vi "arduinoSendCommand.vi"(4 "Wait For Completion":bool=TRUE, 6 "Input Command":string, 7 "error in (no error)":errorcluster, 9 "Input Recieve Log":string, 10 "VISA resource name":refnum<visa-resource-name>) -> (0 "error out":errorcluster, 1 "Command Accepted":bool, 2 "Output Recieve Log":string, 3 "VISA resource name out":refnum<visa-resource-name>)   [LabVIEW 2019]
panel:
  out "Command Rejected":bool
  in  "Wait For Acceptance":bool=TRUE
  out "Command Root":string
  in  "millisecond timer value":u32=200
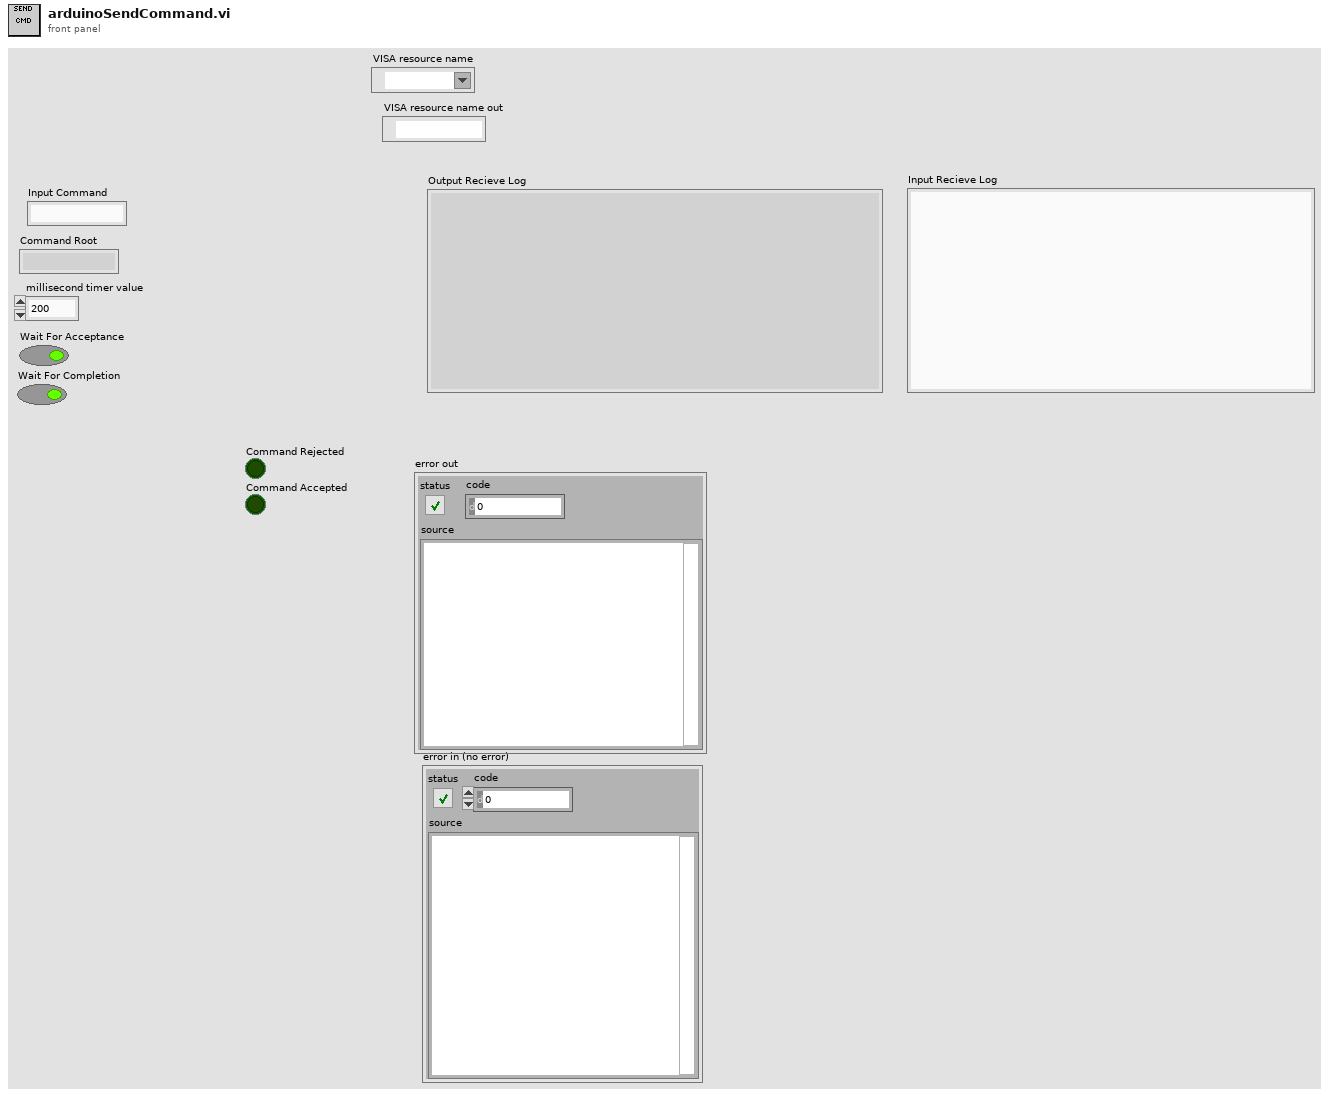
[diagram p1: front panel]
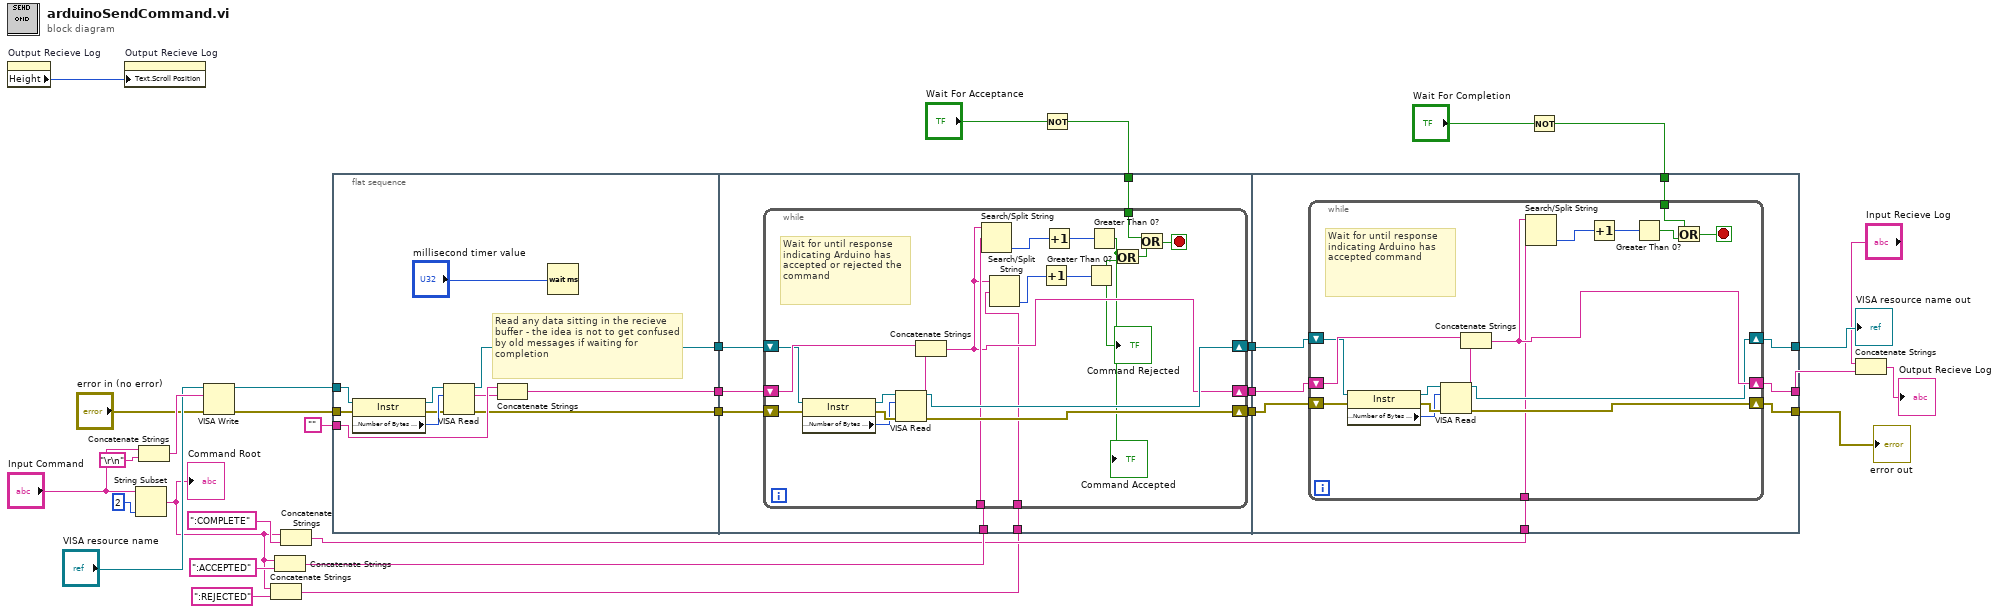
[diagram p0: block diagram]
diagram:
  n1 = property on="Output Recieve Log" class="Str"() -> ("Height"=w30:u32)  [unwired: 2 in, 2 out]
  n2 = property on="Output Recieve Log" class="Str"("Text.Scroll Position"=w30) -> ()  [unwired: 2 in, 2 out]
  n3 = String Subset(string="Input Command", length (rest)=2 ("length (rest)")) -> (substring=w3:string)  [unwired: 1 in]
  "Command Root" <- w3
  n4 = Concatenate Strings("Input Command", "\r\n") -> (w29:string)
  n5 = VISA Write(VISA resource name="VISA resource name", write buffer=w29, error in (no error)="error in (no error)") -> (VISA resource name out=w32:refnum<visa-resource-name>, error out=w31:errorcluster)  [unwired: 1 out]
  n6 = Concatenate Strings(w3, ":REJECTED" ("string")) -> (w1:string)
  n7 = Concatenate Strings(w3, ":ACCEPTED" ("string")) -> (w5:string)
  n8 = Concatenate Strings(w3, ":COMPLETE" ("string")) -> (w4:string)
  n9 = flat-sequence {
    tunnel: w31 -> [w41]
    tunnel: w32 -> [w42]
    tunnel: "" -> [w40]
    tunnel: [w35] -> w27
    tunnel: [w33] -> w13
    tunnel: [w37] -> w12
    tunnel: w27 -> [w50]
    tunnel: w5 -> [w48]
    tunnel: [w52] -> w21
    tunnel: [w51] -> w20
    tunnel: [w49] -> w19
    tunnel: w13 -> [w46]
    tunnel: w12 -> [w47]
    tunnel: w7 -> [w45]
    tunnel: w1 -> [w44]
    tunnel: [w74] -> w10
    tunnel: [w77] -> w23
    tunnel: [w80] -> w24
    tunnel: w21 -> [w81]
    tunnel: w20 -> [w78]
    tunnel: w19 -> [w79]
    tunnel: w6 -> [w76]
    tunnel: w4 -> [w75]
    frame #0 {
      # "Read any data sitting in the recieve buffer - the idea is not to get confused by old messages if waiting for completion"
      n10 = property class="Instr"(reference=w42, error in=w41) -> (reference out=w38:refnum<visa-resource-name>, error out=w34:errorcluster, "Serial Settings:Number of Bytes at Serial Port"=w36:u32)
      n11 = VISA Read(VISA resource name=w38, byte count=w36, error in (no error)=w34) -> (VISA resource name out=w37:refnum<visa-resource-name>, read buffer=w39:string, error out=w33:errorcluster)  [unwired: 1 out]
      n12 = Concatenate Strings(w40, w39) -> (w35:string)
      n13 = Wait (ms)(milliseconds to wait="millisecond timer value") -> ()  [unwired: 1 out]
    }
    frame #1 {
      n14 = while {
        shift-right: [w64] -> w51
        shift-left: w47 -> [w69]
        shift-right: [w65] -> w52
        shift-left: w46 -> [w67]
        shift-right: [w61] -> w49
        shift-left: w50 -> [w72]
        tunnel: w48 -> [w62]
        tunnel: w45 -> [w56]
        tunnel: w44 -> [w60]
        stop <- w53 stop-if-true
        # "Wait for until response indicating Arduino has accepted or rejected the command"
        n15 = property class="Instr"(reference=w69, error in=w67) -> (reference out=w68:refnum<visa-resource-name>, error out=w66:errorcluster, "Serial Settings:Number of Bytes at Serial Port"=w63:u32)
        n16 = VISA Read(VISA resource name=w68, byte count=w63, error in (no error)=w66) -> (VISA resource name out=w64:refnum<visa-resource-name>, read buffer=w73:string, error out=w65:errorcluster)  [unwired: 1 out]
        n17 = Concatenate Strings(w72, w73) -> (w61:string)
        n18 = Search/Split String(string=w61, search string/char (-)=w62) -> (offset of match=w71:i32)  [unwired: 1 in, 2 out]
        n19 = Search/Split String(string=w61, search string/char (-)=w60) -> (offset of match=w59:i32)  [unwired: 1 in, 2 out]
        n20 = Increment(x=w59) -> (x+1=w58:i32)
        n21 = Increment(x=w71) -> (x+1=w70:i32)
        n22 = Greater Than 0?(x=w58) -> (x > 0?=w54:bool)
        "Command Rejected" <- w54
        n23 = Greater Than 0?(x=w70) -> (x > 0?=w57:bool)
        "Command Accepted" <- w57
        n24 = Or(x=w57, y=w54) -> (x .or. y?=w55:bool)
        n25 = Or(x=w56, y=w55) -> (x .or. y?=w53:bool)
      }
    }
    frame #2 {
      n26 = while {
        shift-right: [w86] -> w77
        shift-left: w78 -> [w91]
        shift-right: [w87] -> w80
        shift-left: w81 -> [w89]
        shift-right: [w93] -> w74
        shift-left: w79 -> [w96]
        tunnel: w76 -> [w83]
        tunnel: w75 -> [w82]
        stop <- w92 stop-if-true
        # "Wait for until response indicating Arduino has accepted command"
        n27 = property class="Instr"(reference=w91, error in=w89) -> (reference out=w90:refnum<visa-resource-name>, error out=w88:errorcluster, "Serial Settings:Number of Bytes at Serial Port"=w85:u32)
        n28 = VISA Read(VISA resource name=w90, byte count=w85, error in (no error)=w88) -> (VISA resource name out=w86:refnum<visa-resource-name>, read buffer=w97:string, error out=w87:errorcluster)  [unwired: 1 out]
        n29 = Concatenate Strings(w96, w97) -> (w93:string)
        n30 = Search/Split String(string=w93, search string/char (-)=w82) -> (offset of match=w95:i32)  [unwired: 1 in, 2 out]
        n31 = Increment(x=w95) -> (x+1=w94:i32)
        n32 = Greater Than 0?(x=w94) -> (x > 0?=w84:bool)
        n33 = Or(x=w83, y=w84) -> (x .or. y?=w92:bool)
      }
    }
  }
  n34 = Not(x="Wait For Acceptance") -> (.not. x?=w7:bool)
  n35 = Not(x="Wait For Completion") -> (.not. x?=w6:bool)
  n36 = Concatenate Strings("Input Recieve Log", w10) -> (→"Output Recieve Log":string)
  "error out" <- w24
  "VISA resource name out" <- w23
